vi "PID_controller_06.vi"() -> ()   [LabVIEW 2011]
uses:
  <vilib>/Platform/TimedLoop/XDataNode/nitl_modes.ctl
  <vilib>/Platform/TimedLoop/XDataNode/timing_clust.ctl
  <vilib>/Platform/TimedLoop/XDataNode/wakeup.ctl
  <vilib>/Platform/TimedLoop/XDataNode/XDataNode.xnode
  <vilib>/Platform/TimedLoop/XDataNode/XDNodeRunTimeDep.lvlib
panel:
  out "Idemon":dbl
  out "Inumer":dbl
  out "error(t-t0)":cluster{dbl, "Value":dbl}[](array[cluster])
  out "error":dbl
  out "tStart(s)":dbl
  out "x-y":dbl
  out "S00":dbl
  out "S10":dbl
  out "S20":dbl
  out "S11":dbl
  out "S01":dbl
  out "weight":dbl[](array[numeric])
  in  "# of points to watch":i32
  in  "tSmooth(s)":dbl=-1.0
  out "t0":dbl
  out "error(t)":cluster{dbl, "Value":dbl}[](array[cluster])
  out "error out":errorcluster
  out "first":bool=TRUE
  out "P (torr)":string
  out "XY Graph":cluster{dbl, "Value":dbl}[](graph)
  out "current value":dbl
  in  "stop":bool
  in  "Period (s)":dbl
  out "dValue":dbl
  out "derivative":dbl
  out "integral":dbl
  out "Current angle (deg)":dbl
  in  "Kd":dbl
  in  "Ki":dbl
  in  "Kp":dbl
  out "Current P (torr)":dbl
  in  "Set Point (torr)":dbl
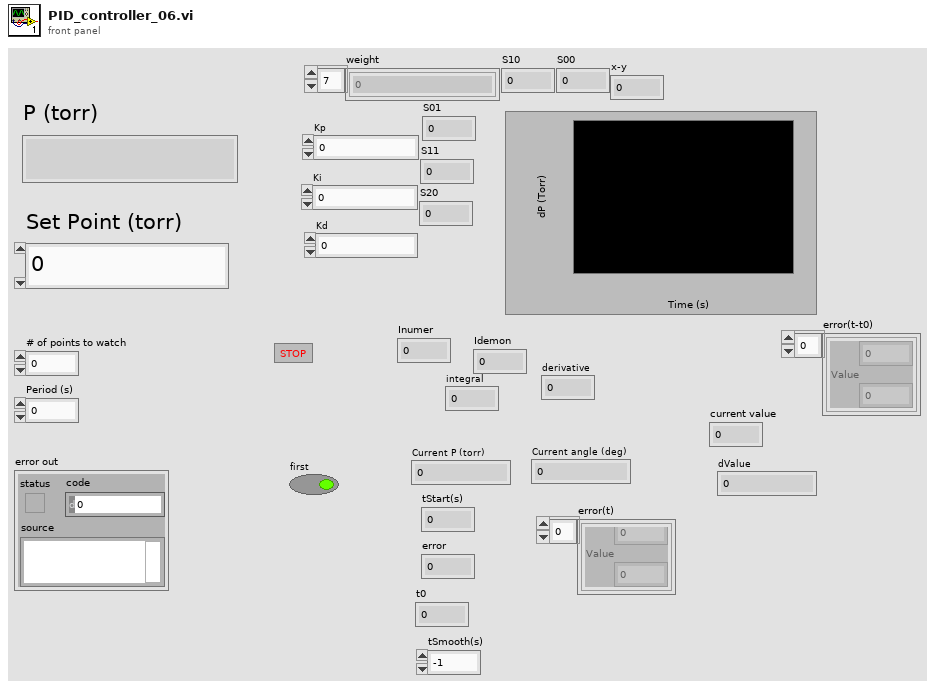
[diagram p1: front panel]
types:
  T1 = typedef "XDNodeRunTimeDep.lvlib/nitl_modes.ctl" = enum32{"No Change", "Process missed periods, maintain original phase", "Discard missed periods, maintain original phase", "Process missed periods, ignore original phase", "Discard missed periods, ignore original phase"}
  T2 = typedef "XDNodeRunTimeDep.lvlib/timing_clust.ctl" = cluster{"Expected End [f-1]":u64, "Actual End [f-1]":u64, "Finished Late? [f-1]":bool, "Expected End [i-1]":u64, "Actual End [i-1]":u64, "Finished Late? [i-1]":bool, "Expected Start [i]":u64, "Actual Start [i]":u64, "Expected Start [f]":u64, "Actual Start [f]":u64, "Source Name":string, "Structure Name":string, "Period":i64, "Deadline":i64, "Offset":i64, "Start":i64, "Priority":i32, "Timeout":i32, "Mode":T1, "Wakeup Reason":T3, "Error":errorcluster, "Source Type":string, "Secondary Source Type":string, "Global End Time":u64, "Global Start Time":u64, "Frame Duration":u64, "Iteration Duration":u64, "Assigned CPU":i32, "I/O Scan Engine Mode":u32}
  T3 = typedef "XDNodeRunTimeDep.lvlib/wakeup.ctl" = enum32{"Normal", "Aborted", "Asynchronous wakeup", "Timing source error", "Timed loop error", "Timeout"}
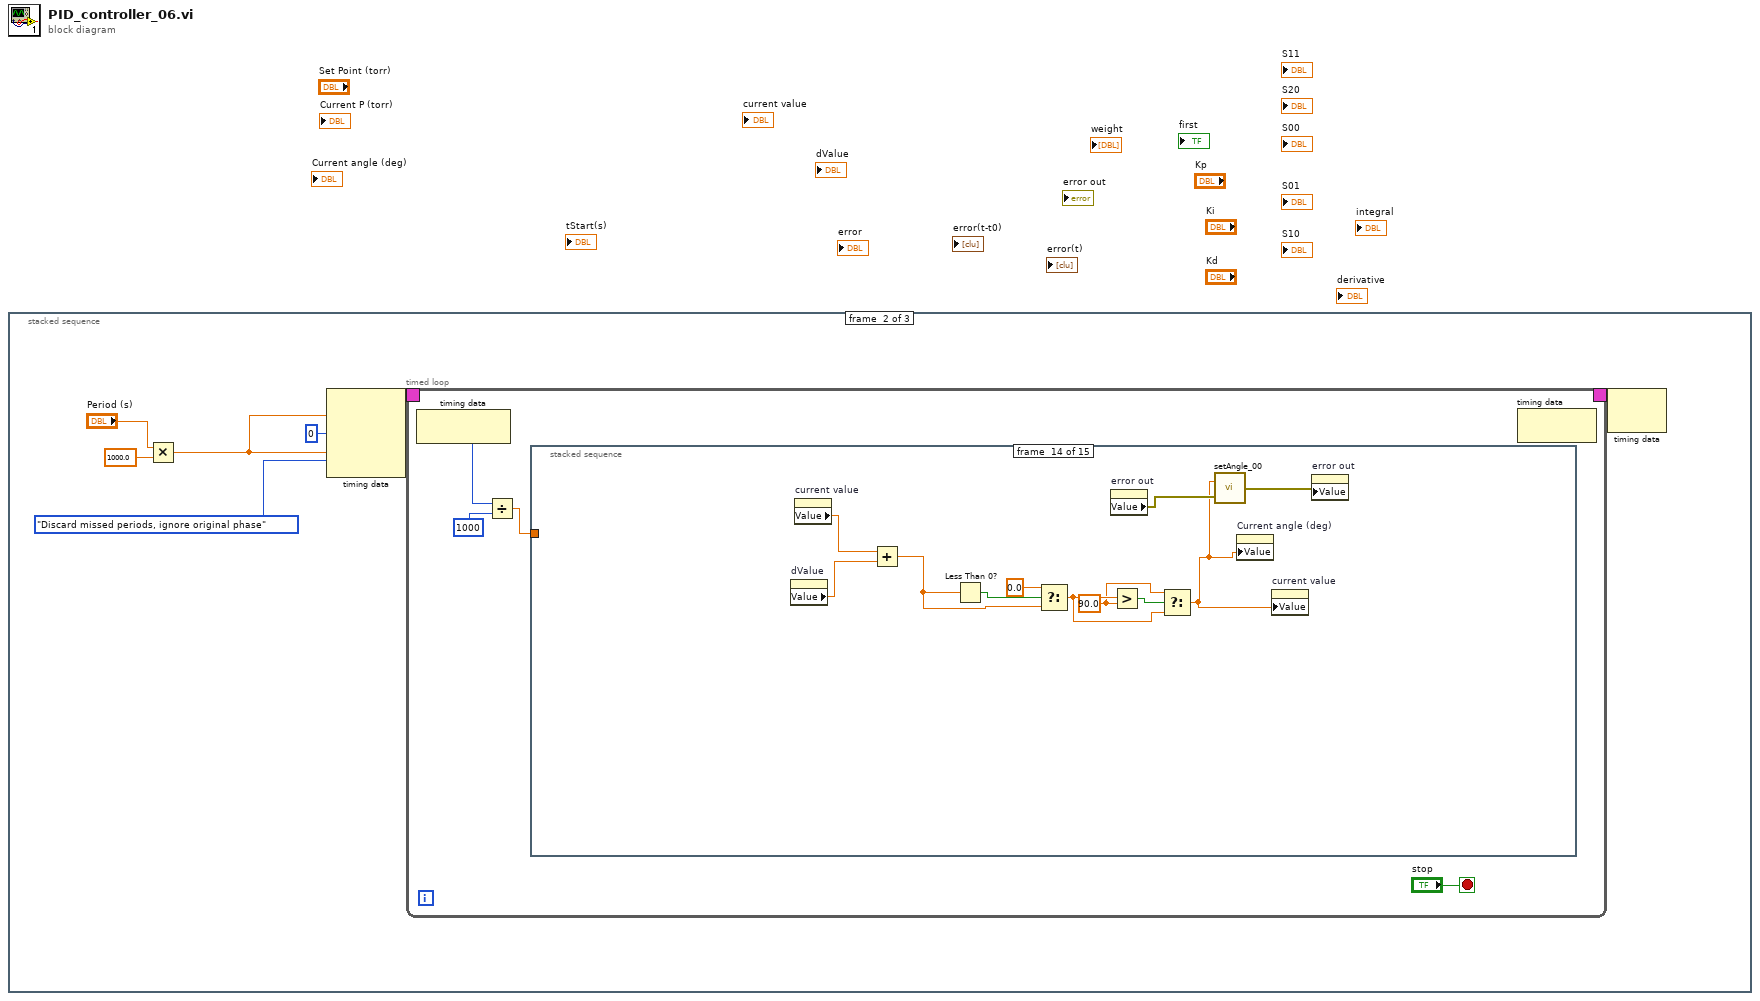
[diagram p0: block diagram]
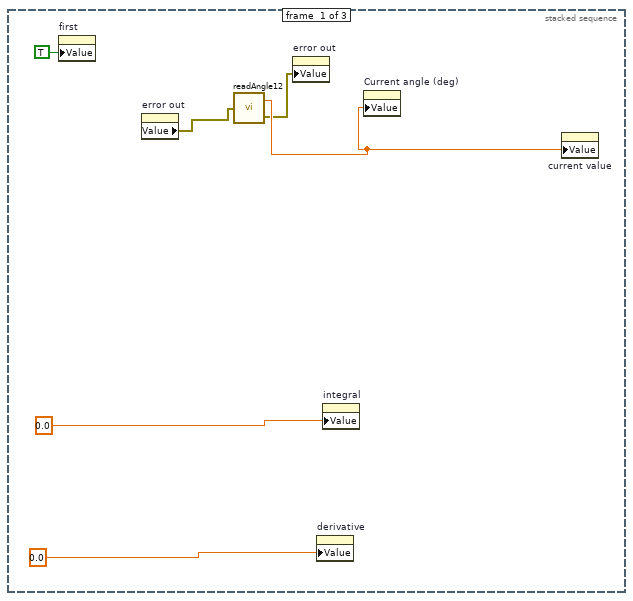
[diagram p2: hidden frame]
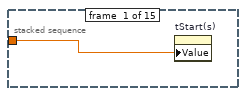
[diagram p3: hidden frame]
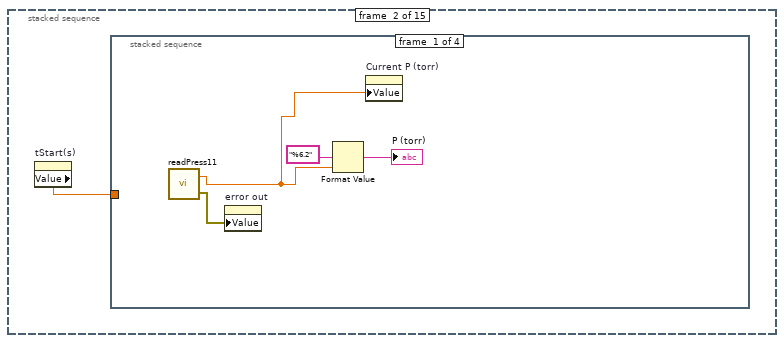
[diagram p4: hidden frame]
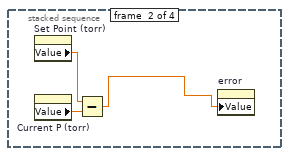
[diagram p5: hidden frame]
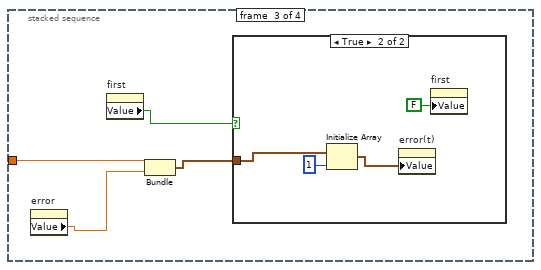
[diagram p6: hidden frame]
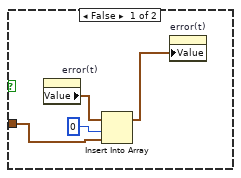
[diagram p7: hidden frame]
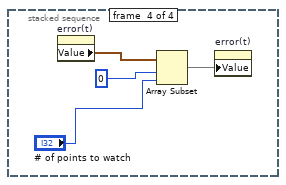
[diagram p8: hidden frame]
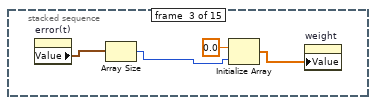
[diagram p9: hidden frame]
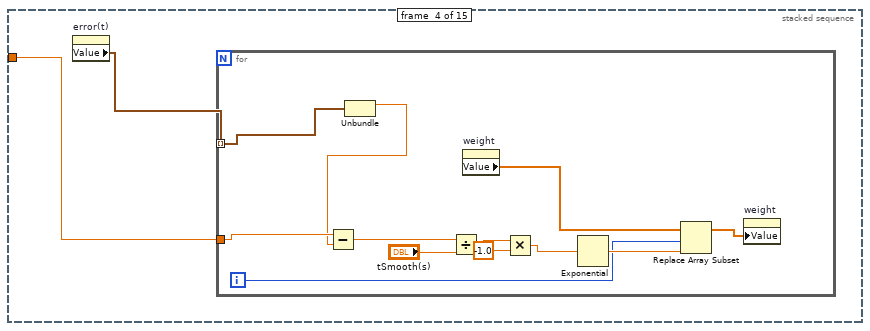
[diagram p10: hidden frame]
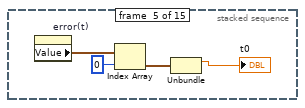
[diagram p11: hidden frame]
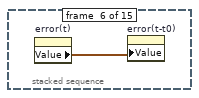
[diagram p12: hidden frame]
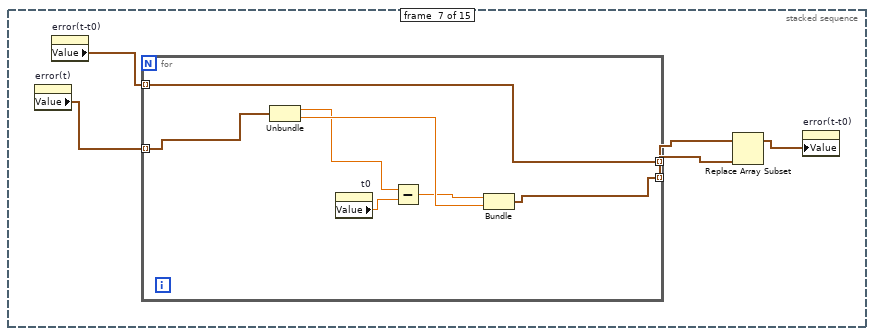
[diagram p13: hidden frame]
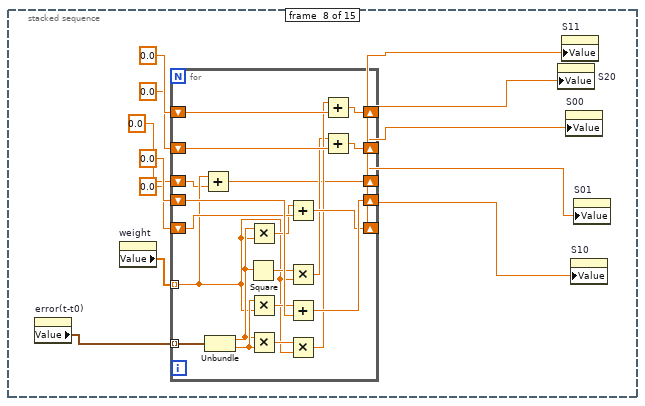
[diagram p14: hidden frame]
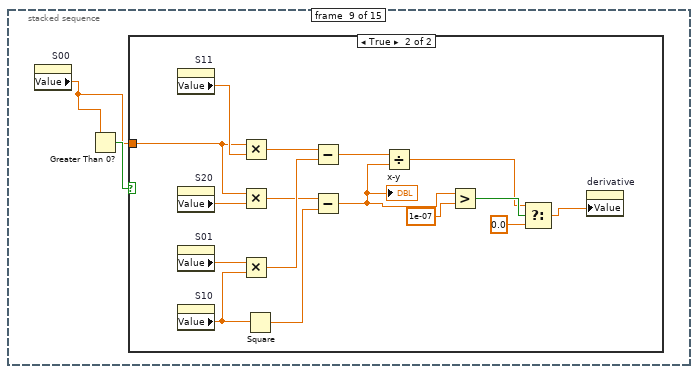
[diagram p15: hidden frame]
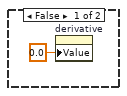
[diagram p16: hidden frame]
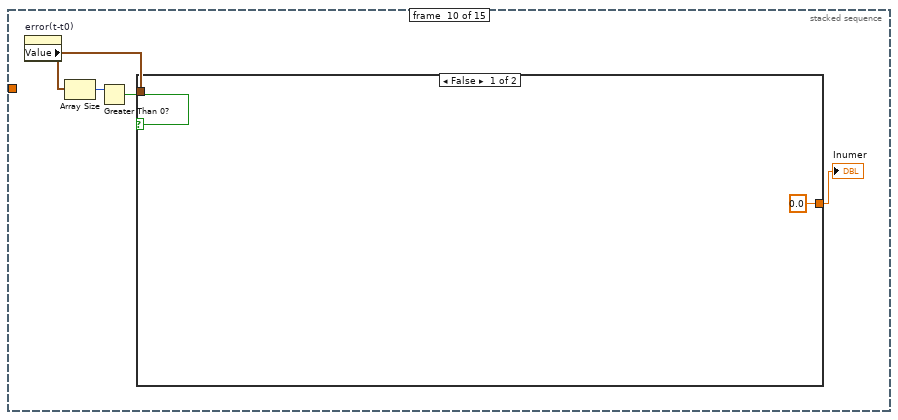
[diagram p17: hidden frame]
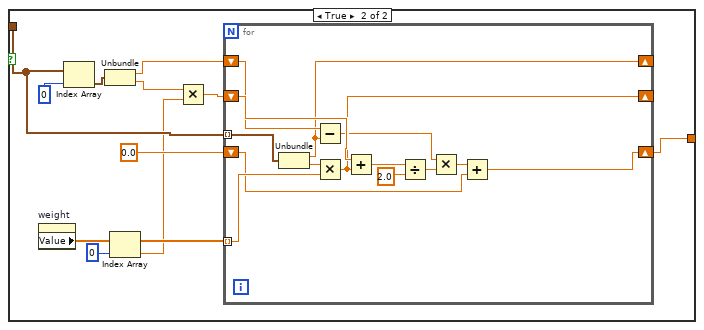
[diagram p18: hidden frame]
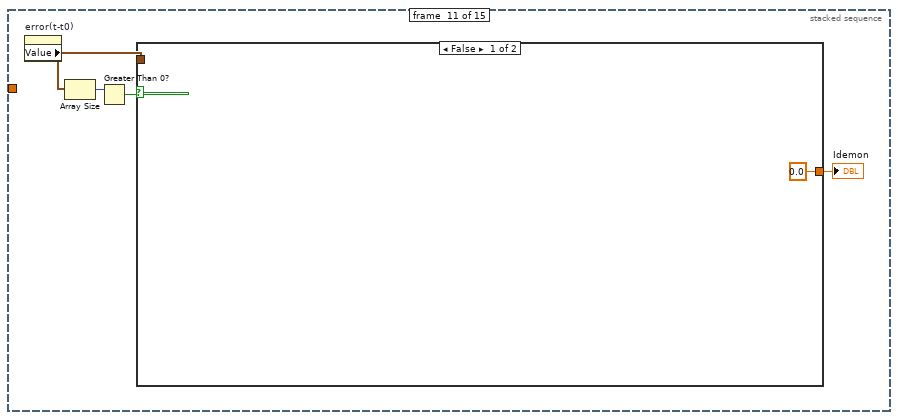
[diagram p19: hidden frame]
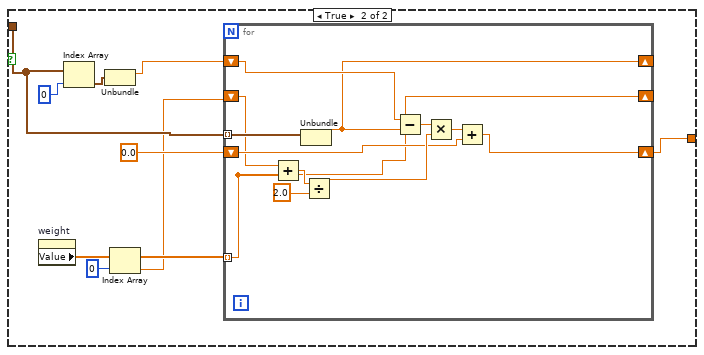
[diagram p20: hidden frame]
diagram:
  n1 = stacked-sequence {
    frame #0 {
      n2 = property on="first" class="Bool (strict)"("Value"=TRUE ("first")) -> ()  [unwired: 2 in, 2 out]
      n3 = property on="error out" class="Clust (strict)"() -> ("Value"=w2:errorcluster)  [unwired: 2 in, 2 out]
      n4 = call "readAngle12.vi"("error in"=w2) -> ("angle"=w3:dbl, "error out"=w1:errorcluster)
      n5 = property on="error out" class="Clust (strict)"("Value"=w1) -> ()  [unwired: 2 in, 2 out]
      n6 = property on="derivative" class="DigNum (strict)"("Value"=0.0 ("derivative")) -> ()  [unwired: 2 in, 2 out]
      n7 = property on="integral" class="DigNum (strict)"("Value"=0.0 ("integral")) -> ()  [unwired: 2 in, 2 out]
      n8 = property on="Current angle (deg)" class="DigNum (strict)"("Value"=w3) -> ()  [unwired: 2 in, 2 out]
      n9 = property on="current value" class="DigNum (strict)"("Value"=w3) -> ()  [unwired: 2 in, 2 out]
    }
    frame #1 {
      n10 = Multiply(x="Period (s)", y=1000.0) -> (x*y=w8:dbl)
      n11 = node-c288(w8, i64 0 ("Offset"), w8, nitl_modes."Discard missed periods, ignore original phase" ("Mode")) -> (w13:T2)
      n12 = timed-loop {
        timing: w13 -> [_]
        timing-out: [_] -> w12
        stop <- "stop" stop-if-true
        n13 = node-c288() -> (w14:i64)  [unwired: 1 in]
        n14 = Divide(x=w14, y=i64 1000) -> (x/y=w15:dbl)
        n15 = stacked-sequence {
          tunnel: w15 -> [w18 _ _ w47 _ _ _ _ _ _ _ _ _ _ _]
          frame #0 {
            n16 = property on="tStart(s)" class="DigNum (strict)"("Value"=w18) -> ()  [unwired: 2 in, 2 out]
          }
          frame #1 {
            n17 = property on="tStart(s)" class="DigNum (strict)"() -> ("Value"=w19:dbl)  [unwired: 2 in, 2 out]
            n18 = stacked-sequence {
              tunnel: w19 -> [_ _ w29 _]
              frame #0 {
                n19 = call "readPress11.vi"() -> ("P"=w21:dbl, "error out"=w20:errorcluster)  [unwired: 1 in]
                n20 = property on="error out" class="Clust (strict)"("Value"=w20) -> ()  [unwired: 2 in, 2 out]
                n21 = Format Value(format string="%6.2", value (0)=w21) -> (output string=→"P (torr)":string)  [unwired: 1 in]
                n22 = property on="Current P (torr)" class="DigNum (strict)"("Value"=w21) -> ()  [unwired: 2 in, 2 out]
              }
              frame #1 {
                n23 = property on="Set Point (torr)" class="DigNum (strict)"() -> ("Value"=w25:dbl)  [unwired: 2 in, 2 out]
                n24 = property on="Current P (torr)" class="DigNum (strict)"() -> ("Value"=w26:dbl)  [unwired: 2 in, 2 out]
                n25 = Subtract(x=w25, y=w26) -> (x-y=w24:dbl)
                n26 = property on="error" class="DigNum (strict)"("Value"=w24) -> ()  [unwired: 2 in, 2 out]
              }
              frame #2 {
                n27 = property on="error" class="DigNum (strict)"() -> ("Value"=w27:dbl)  [unwired: 2 in, 2 out]
                n28 = property on="first" class="Bool (strict)"() -> ("Value"=w30:bool)  [unwired: 2 in, 2 out]
                n29 = Bundle("Value"=w29, "Value"=w27) -> (w28:cluster{"Value":dbl, "Value":dbl})  [unwired: 1 in]
                n30 = case shown="True" w30 {
                  tunnel: w28 -> [w32 w37]
                  frame False {
                    n31 = property on="error(t)" class="Arr (strict)"() -> ("Value"=w33:cluster{dbl, "Value":dbl}[])  [unwired: 2 in, 2 out]
                    n32 = Insert Into Array(array=w33, index=0, new element=w32) -> (w31:cluster{dbl, "Value":dbl}[])
                    n33 = property on="error(t)" class="Arr (strict)"("Value"=w31) -> ()  [unwired: 2 in, 2 out]
                  }
                  frame True {
                    n34 = Initialize Array(w37, 1 ("dimension size")) -> (w35:cluster{"Value":dbl, "Value":dbl}[])
                    n35 = property on="error(t)" class="Arr (strict)"("Value"=w35) -> ()  [unwired: 2 in, 2 out]
                    n36 = property on="first" class="Bool (strict)"("Value"=FALSE ("first")) -> ()  [unwired: 2 in, 2 out]
                  }
                }
              }
              frame #3 {
                n37 = property on="error(t)" class="Arr (strict)"() -> ("Value"=w40:cluster{dbl, "Value":dbl}[])  [unwired: 2 in, 2 out]
                n38 = Array Subset(array=w40, index=0, length="# of points to watch") -> (w42:cluster{dbl, "Value":dbl}[])
                n39 = property on="error(t)" class="Arr (strict)"("Value"=w42) -> ()  [unwired: 2 in, 2 out]
              }
            }
          }
          frame #2 {
            n40 = property on="error(t)" class="Arr (strict)"() -> ("Value"=w46:cluster{dbl, "Value":dbl}[])  [unwired: 2 in, 2 out]
            n41 = Array Size(array=w46) -> (size(s)=w44:i32)
            n42 = Initialize Array(0.0 ("element"), w44) -> (w43:dbl[])
            n43 = property on="weight" class="Arr (strict)"("Value"=w43) -> ()  [unwired: 2 in, 2 out]
          }
          frame #3 {
            n44 = property on="error(t)" class="Arr (strict)"() -> ("Value"=w48:cluster{dbl, "Value":dbl}[])  [unwired: 2 in, 2 out]
            n45 = for {
              tunnel: w48 -> [w60] mode=indexing
              tunnel: w47 -> [w59]
              i -> [w55]
              n46 = Unbundle(w60) -> (w58:dbl)  [unwired: 1 out]
              n47 = Subtract(x=w59, y=w58) -> (x-y=w53:dbl)
              n48 = Divide(x=w53, y="tSmooth(s)") -> (x/y=w51:dbl)
              n49 = property on="weight" class="Arr (strict)"() -> ("Value"=w56:dbl[])  [unwired: 2 in, 2 out]
              n50 = Multiply(x=w51, y=-1.0) -> (x*y=w49:dbl)
              n51 = Exponential(1:w49) -> (0:w57:dbl)
              n52 = Replace Array Subset(array=w56, new element=w57, index=w55) -> (w54:dbl[])
              n53 = property on="weight" class="Arr (strict)"("Value"=w54) -> ()  [unwired: 2 in, 2 out]
            }
          }
          frame #4 {
            n54 = property on="error(t)" class="Arr (strict)"() -> ("Value"=w64:cluster{dbl, "Value":dbl}[])  [unwired: 2 in, 2 out]
            n55 = Index Array(array=w64, index=0) -> (element=w62:cluster{dbl, "Value":dbl})
            n56 = Unbundle(w62) -> (→"t0":dbl)  [unwired: 1 out]
          }
          frame #5 {
            n57 = property on="error(t)" class="Arr (strict)"() -> ("Value"=w65:cluster{dbl, "Value":dbl}[])  [unwired: 2 in, 2 out]
            n58 = property on="error(t-t0)" class="Arr (strict)"("Value"=w65) -> ()  [unwired: 2 in, 2 out]
          }
          frame #6 {
            n59 = property on="error(t)" class="Arr (strict)"() -> ("Value"=w70:cluster{dbl, "Value":dbl}[])  [unwired: 2 in, 2 out]
            n60 = property on="error(t-t0)" class="Arr (strict)"() -> ("Value"=w68:cluster{dbl, "Value":dbl}[])  [unwired: 2 in, 2 out]
            n61 = for {
              tunnel: w70 -> [w73] mode=indexing
              tunnel: [w72] -> w69 mode=indexing
              tunnel: w68 -> [w71] mode=indexing
              tunnel: [w71] -> w67 mode=indexing
              n62 = Unbundle(w73) -> (w74:dbl, "Value"=w76:dbl)
              n63 = property on="t0" class="DigNum (strict)"() -> ("Value"=w77:dbl)  [unwired: 2 in, 2 out]
              n64 = Subtract(x=w74, y=w77) -> (x-y=w75:dbl)
              n65 = Bundle(w75, "Value"=w76) -> (w72:cluster{dbl, "Value":dbl})  [unwired: 1 in]
            }
            n66 = Replace Array Subset(array=w67, new element=w69) -> (w66:cluster{dbl, "Value":dbl}[])  [unwired: 1 in]
            n67 = property on="error(t-t0)" class="Arr (strict)"("Value"=w66) -> ()  [unwired: 2 in, 2 out]
          }
          frame #7 {
            n68 = property on="error(t-t0)" class="Arr (strict)"() -> ("Value"=w78:cluster{dbl, "Value":dbl}[])  [unwired: 2 in, 2 out]
            n69 = property on="weight" class="Arr (strict)"() -> ("Value"=w85:dbl[])  [unwired: 2 in, 2 out]
            n70 = for {
              tunnel: w78 -> [w105] mode=indexing
              shift-right: [w106] -> w80
              shift-left: 0.0 -> [w109]
              shift-right: [w102] -> w83
              shift-left: 0.0 -> [w108]
              shift-right: [w101] -> w82
              shift-left: 0.0 -> [w107]
              shift-right: [w103] -> w79
              shift-left: 0.0 -> [w104]
              tunnel: w85 -> [w92] mode=indexing
              shift-right: [w90] -> w81
              shift-left: 0.0 -> [w91]
              n71 = Add(x=w92, y=w91) -> (x+y=w90:dbl)
              n72 = Unbundle(w105) -> (w94:dbl, "Value"=w100:dbl)
              n73 = Square(x=w94) -> (x^2=w96:dbl)
              n74 = Multiply(x=w94, y=w92) -> (x*y=w93:dbl)
              n75 = Multiply(x=w100, y=w92) -> (x*y=w99:dbl)
              n76 = Multiply(x=w94, y=w100) -> (x*y=w98:dbl)
              n77 = Add(x=w93, y=w104) -> (x+y=w103:dbl)
              n78 = Multiply(x=w96, y=w92) -> (x*y=w95:dbl)
              n79 = Add(x=w99, y=w109) -> (x+y=w106:dbl)
              n80 = Multiply(x=w98, y=w92) -> (x*y=w97:dbl)
              n81 = Add(x=w97, y=w108) -> (x+y=w102:dbl)
              n82 = Add(x=w95, y=w107) -> (x+y=w101:dbl)
            }
            n83 = property on="S20" class="DigNum (strict)"("Value"=w82) -> ()  [unwired: 2 in, 2 out]
            n84 = property on="S11" class="DigNum (strict)"("Value"=w83) -> ()  [unwired: 2 in, 2 out]
            n85 = property on="S00" class="DigNum (strict)"("Value"=w81) -> ()  [unwired: 2 in, 2 out]
            n86 = property on="S10" class="DigNum (strict)"("Value"=w79) -> ()  [unwired: 2 in, 2 out]
            n87 = property on="S01" class="DigNum (strict)"("Value"=w80) -> ()  [unwired: 2 in, 2 out]
          }
          frame #8 {
            n88 = property on="S00" class="DigNum (strict)"() -> ("Value"=w110:dbl)  [unwired: 2 in, 2 out]
            n89 = Greater Than 0?(x=w110) -> (x > 0?=w111:bool)
            n90 = case shown="True" w111 {
              tunnel: w110 -> [_ w120]
              frame False {
                n91 = property on="derivative" class="DigNum (strict)"("Value"=0.0 ("derivative")) -> ()  [unwired: 2 in, 2 out]
              }
              frame True {
                n92 = property on="S11" class="DigNum (strict)"() -> ("Value"=w122:dbl)  [unwired: 2 in, 2 out]
                n93 = property on="S20" class="DigNum (strict)"() -> ("Value"=w121:dbl)  [unwired: 2 in, 2 out]
                n94 = property on="S01" class="DigNum (strict)"() -> ("Value"=w119:dbl)  [unwired: 2 in, 2 out]
                n95 = property on="S10" class="DigNum (strict)"() -> ("Value"=w123:dbl)  [unwired: 2 in, 2 out]
                n96 = Multiply(x=w120, y=w122) -> (x*y=w128:dbl)
                n97 = Multiply(x=w120, y=w121) -> (x*y=w126:dbl)
                n98 = Multiply(x=w119, y=w123) -> (x*y=w127:dbl)
                n99 = Square(x=w123) -> (x^2=w125:dbl)
                n100 = Subtract(x=w128, y=w127) -> (x-y=w124:dbl)
                n101 = Subtract(x=w126, y=w125) -> (x-y=w118:dbl)
                "x-y" <- w118
                n102 = Divide(x=w124, y=w118) -> (x/y=w114:dbl)
                n103 = Greater?(x=w118, y=1e-07) -> (0:w116:bool)
                n104 = Select(t=w114, s=w116, f=0.0) -> (s? t:f=w115:dbl)
                n105 = property on="derivative" class="DigNum (strict)"("Value"=w115) -> ()  [unwired: 2 in, 2 out]
              }
            }
          }
          frame #9 {
            n106 = property on="error(t-t0)" class="Arr (strict)"() -> ("Value"=w130:cluster{dbl, "Value":dbl}[])  [unwired: 2 in, 2 out]
            n107 = Array Size(array=w130) -> (size(s)=w132:i32)
            n108 = Greater Than 0?(x=w132) -> (x > 0?=w131:bool)
            n109 = case shown="False" w131 {
              tunnel: [0.0 w144] -> w129
              tunnel: w130 -> [_ w142]
              frame False {
              }
              frame True {
                n110 = property on="weight" class="Arr (strict)"() -> ("Value"=w138:dbl[])  [unwired: 2 in, 2 out]
                n111 = Index Array(array=w142, index=0) -> (element=w140:cluster{dbl, "Value":dbl})
                n112 = Unbundle(w140) -> (w139:dbl, "Value"=w136:dbl)
                n113 = Index Array(array=w138, index=0) -> (element=w135:dbl)
                n114 = Multiply(x=w136, y=w135) -> (x*y=w134:dbl)
                n115 = for {
                  tunnel: w142 -> [w158] mode=indexing
                  shift-right: [w152] -> _
                  shift-left: w139 -> [w153]
                  tunnel: w138 -> [w154] mode=indexing
                  shift-right: [w145] -> w144
                  shift-left: 0.0 -> [w146]
                  shift-right: [w150] -> _
                  shift-left: w134 -> [w155]
                  n116 = Unbundle(w158) -> (w152:dbl, "Value"=w151:dbl)
                  n117 = Subtract(x=w153, y=w152) -> (x-y=w149:dbl)
                  n118 = Multiply(x=w151, y=w154) -> (x*y=w150:dbl)
                  n119 = Add(x=w155, y=w150) -> (x+y=w157:dbl)
                  n120 = Divide(x=w157, y=2.0) -> (x/y=w148:dbl)
                  n121 = Multiply(x=w149, y=w148) -> (x*y=w147:dbl)
                  n122 = Add(x=w147, y=w146) -> (x+y=w145:dbl)
                }
              }
            }
            "Inumer" <- w129
          }
          frame #10 {
            n123 = property on="error(t-t0)" class="Arr (strict)"() -> ("Value"=w160:cluster{dbl, "Value":dbl}[])  [unwired: 2 in, 2 out]
            n124 = Array Size(array=w160) -> (size(s)=w162:i32)
            n125 = Greater Than 0?(x=w162) -> (x > 0?=w161:bool)
            n126 = case shown="False" w161 {
              tunnel: [0.0 w172] -> w159
              tunnel: w160 -> [_ w170]
              frame False {
              }
              frame True {
                n127 = property on="weight" class="Arr (strict)"() -> ("Value"=w166:dbl[])  [unwired: 2 in, 2 out]
                n128 = Index Array(array=w170, index=0) -> (element=w168:cluster{dbl, "Value":dbl})
                n129 = Unbundle(w168) -> (w167:dbl)  [unwired: 1 out]
                n130 = Index Array(array=w166, index=0) -> (element=w164:dbl)
                n131 = for {
                  tunnel: w170 -> [w184] mode=indexing
                  shift-right: [w180] -> _
                  shift-left: w167 -> [w181]
                  tunnel: w166 -> [w174] mode=indexing
                  shift-right: [w175] -> w172
                  shift-left: 0.0 -> [w176]
                  shift-right: [w174] -> _
                  shift-left: w164 -> [w173]
                  n132 = Add(x=w173, y=w174) -> (x+y=w183:dbl)
                  n133 = Unbundle(w184) -> (w180:dbl)  [unwired: 1 out]
                  n134 = Divide(x=w183, y=2.0) -> (x/y=w178:dbl)
                  n135 = Subtract(x=w181, y=w180) -> (x-y=w179:dbl)
                  n136 = Multiply(x=w179, y=w178) -> (x*y=w177:dbl)
                  n137 = Add(x=w177, y=w176) -> (x+y=w175:dbl)
                }
              }
            }
            "Idemon" <- w159
          }
          frame #11 {
            n138 = property on="Idemon" class="DigNum (strict)"() -> ("Value"=w185:dbl)  [unwired: 2 in, 2 out]
            n139 = property on="Inumer" class="DigNum (strict)"() -> ("Value"=w186:dbl)  [unwired: 2 in, 2 out]
            n140 = Divide(x=w186, y=w185) -> (x/y=w189:dbl)
            n141 = Greater Than 0?(x=w185) -> (x > 0?=w190:bool)
            n142 = Select(t=w189, s=w190, f=0.0) -> (s? t:f=w187:dbl)
            n143 = property on="integral" class="DigNum (strict)"("Value"=w187) -> ()  [unwired: 2 in, 2 out]
          }
          frame #12 {
            n144 = property on="error" class="DigNum (strict)"() -> ("Value"=w191:dbl)  [unwired: 2 in, 2 out]
            n145 = property on="Kp" class="DigNum (strict)"() -> ("Value"=w201:dbl)  [unwired: 2 in, 2 out]
            n146 = property on="integral" class="DigNum (strict)"() -> ("Value"=w199:dbl)  [unwired: 2 in, 2 out]
            n147 = property on="derivative" class="DigNum (strict)"() -> ("Value"=w197:dbl)  [unwired: 2 in, 2 out]
            n148 = property on="Ki" class="DigNum (strict)"() -> ("Value"=w200:dbl)  [unwired: 2 in, 2 out]
            n149 = property on="Kd" class="DigNum (strict)"() -> ("Value"=w198:dbl)  [unwired: 2 in, 2 out]
            n150 = Multiply(x=w198, y=w197) -> (x*y=w194:dbl)
            n151 = Multiply(x=w200, y=w199) -> (x*y=w195:dbl)
            n152 = Multiply(x=w201, y=w191) -> (x*y=w196:dbl)
            n153 = Add(x=w196, y=w195) -> (x+y=w193:dbl)
            n154 = Add(x=w193, y=w194) -> (x+y=w192:dbl)
            n155 = property on="dValue" class="DigNum (strict)"("Value"=w192) -> ()  [unwired: 2 in, 2 out]
          }
          frame #13 {
            w203 = 90.0 ("y")
            n156 = property on="dValue" class="DigNum (strict)"() -> ("Value"=w211:dbl)  [unwired: 2 in, 2 out]
            n157 = property on="current value" class="DigNum (strict)"() -> ("Value"=w212:dbl)  [unwired: 2 in, 2 out]
            n158 = Add(x=w212, y=w211) -> (x+y=w204:dbl)
            n159 = Less Than 0?(x=w204) -> (x < 0?=w208:bool)
            n160 = Select(t=0.0, s=w208, f=w204) -> (s? t:f=w205:dbl)
            n161 = property on="error out" class="Clust (strict)"() -> ("Value"=w210:errorcluster)  [unwired: 2 in, 2 out]
            n162 = Greater?(x=w205, y=w203) -> (0:w206:bool)
            n163 = Select(t=w203, s=w206, f=w205) -> (s? t:f=w202:dbl)
            n164 = call "setAngle_00.vi"("error in (no error)"=w210, "Angle (deg)"=w202) -> ("error out"=w209:errorcluster)
            n165 = property on="Current angle (deg)" class="DigNum (strict)"("Value"=w202) -> ()  [unwired: 2 in, 2 out]
            n166 = property on="current value" class="DigNum (strict)"("Value"=w202) -> ()  [unwired: 2 in, 2 out]
            n167 = property on="error out" class="Clust (strict)"("Value"=w209) -> ()  [unwired: 2 in, 2 out]
          }
          frame #14 {
            n168 = property on="error(t-t0)" class="Arr (strict)"() -> ("Value"=→"XY Graph":cluster{dbl, "Value":dbl}[])  [unwired: 2 in, 2 out]
          }
        }
        n169 = node-c288() -> ()  [unwired: 1 in, 1 out]
      }
      n170 = node-c288(w12) -> ()  [unwired: 1 out]
    }
    frame #2 {
      n171 = call "WriteAdaptorr03.vi"("string to write"="D5") -> ()  [unwired: 1 in, 1 out]
    }
  }
